vi "EV3_Python.vi"() -> ()   [LabVIEW 2018]
panel:
  in  "Tab Control":enum32{"Connect", "Python"}(tab)
  in  "EV3 IP Address":string="169.254.90.224"
  in  "Ping":bool
  out "Success?":bool
  in  "SSH":bool
  out "SSH Success?":bool
  in  "Script":string="from pybricks import ev3brick as brick\nfrom pybricks.ev3devices import Motor, TouchSensor, ColorSensor,InfraredSensor, UltrasonicSensor, GyroSensor\n\nfrom pybricks.parameters import Port, Stop, Direction, Button, Color, Align\n\nfrom pybricks.tools import wait, StopWatch\n\nexample_motor = Motor (Port.A)"
  out "Console":string
  in  "Help Button":bool
  in  "Run DIrect":bool
  in  "Ctrl C":bool
  in  "Done":bool
  # "Steps:\nGet EV3Dev running\n0. go to https://education.lego.com/en-us/support/mindstorms-ev3/python-for-ev3\n1. burn an SDCard\n2. turn on EV3 with card in\n3. connect to PC\n4. go to Wireless and Networks\n       to All Network Cinnections\n5. select Wired\n6. copy IP address (upper left) \n\nGet Labview running\n7. pip install paramiko  (SSH)\n8. Run this program\n9. hit ping to make sure it is there\n10. hit SSH In\n11. start python"
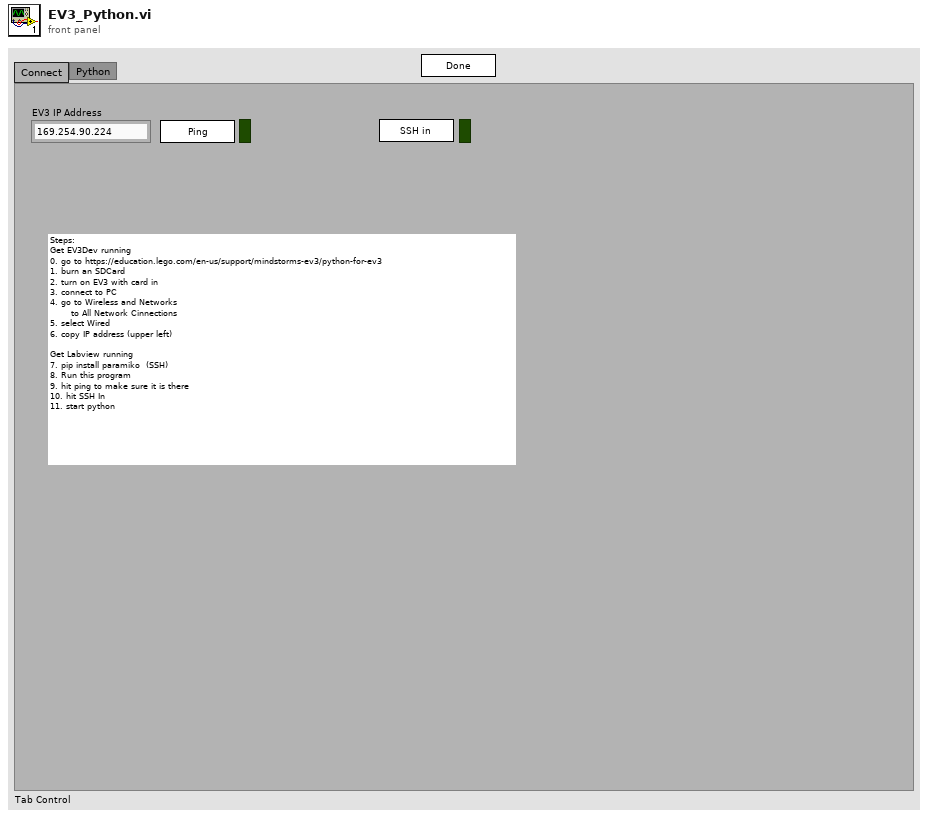
[diagram p1: front panel]
types:
  T1 = typedef "eventvkey.ctl" = enum16{"ASCII", "Enter", "Return", "Shift", "Ctrl", "Alt", "Cmd", "Opt", "Caps", "NumLock", "Clear", "Break", "Up", "Down", "Left", "Right", "Insert", "Delete", "Home", "End", "PageUp", "PageDown", "Escape", "Help", "Pause", "ScrollLock", "F1", "F2", "F3", "F4", "F5", "F6", "F7", "F8", "F9", "F10", "F11", "F12", "F13", "F14", "F15", "F16", "F17", "F18", "F19", "F20", "F21", "F22", "F23", "F24", "Play", "VolumeUp", "VolumeDown", "Mute", "Two Byte Char"}
  T2 = cluster{"Shift":bool, "Ctrl":bool, "Alt":bool, "Cmd":bool, "Opt":bool}
  T3 = cluster{"Char":i16, "VKey":T1, "ScanCode":i16, "Mods":cluster{"Num Pad":bool, "Menu Key":bool}, "PlatMods":cluster{"Shift":bool, "Ctrl":bool, "Alt":bool, "Cmd":bool, "Opt":bool}, "FocusObj":refnum<vi>}
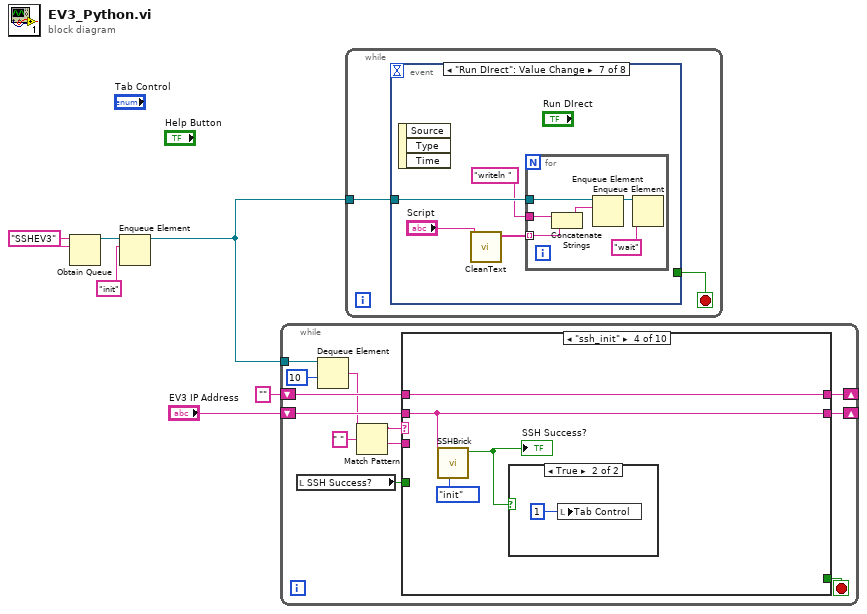
[diagram p0: block diagram]
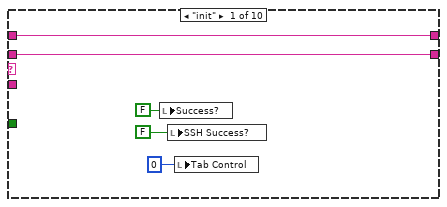
[diagram p2: hidden frame]
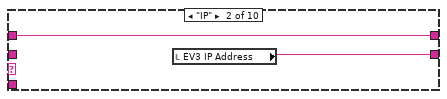
[diagram p3: hidden frame]
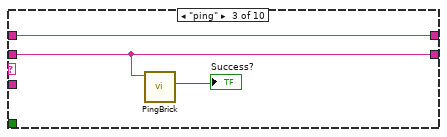
[diagram p4: hidden frame]
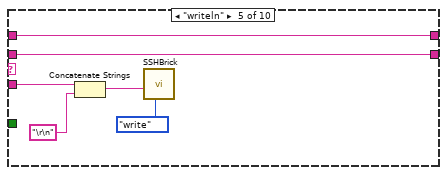
[diagram p6: hidden frame]
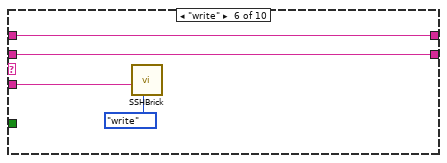
[diagram p7: hidden frame]
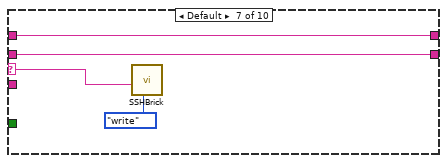
[diagram p8: hidden frame]
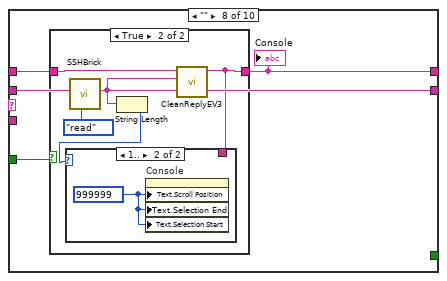
[diagram p9: hidden frame]
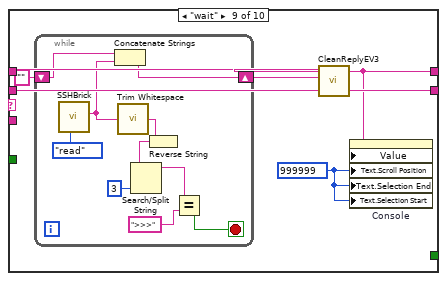
[diagram p12: hidden frame]
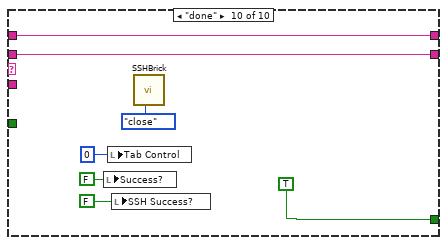
[diagram p13: hidden frame]
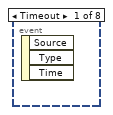
[diagram p14: hidden frame]
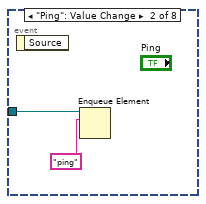
[diagram p15: hidden frame]
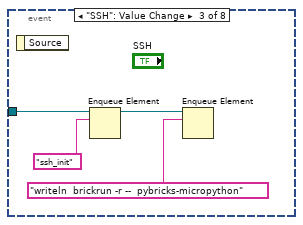
[diagram p16: hidden frame]
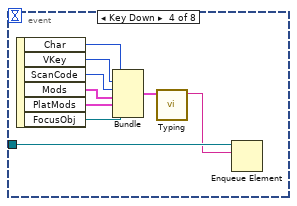
[diagram p17: hidden frame]
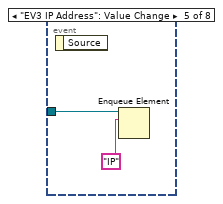
[diagram p18: hidden frame]
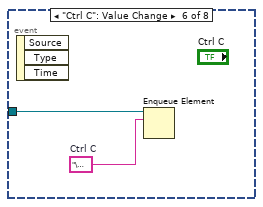
[diagram p19: hidden frame]
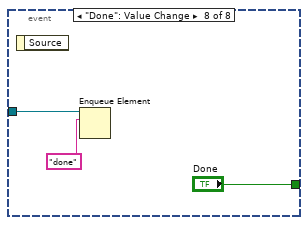
[diagram p20: hidden frame]
diagram:
  w4 = "SSHEV3" ("name (unnamed)")
  n1 = Obtain Queue(name (unnamed)=w4, element data type=w4) -> (queue out=w6:refnum<queue>)  [unwired: 3 in, 2 out]
  n2 = Enqueue Element(queue=w6, element="init") -> (queue out=w3:refnum<queue>)  [unwired: 2 in, 2 out]
  n3 = while {
    tunnel: w3 -> [w18]
    shift-right: [w15] -> _
    shift-left: "EV3 IP Address" -> [w16]
    shift-right: [w13] -> _
    shift-left: "" -> [w14]
    stop <- w17 stop-if-true
    n4 = local read "SSH Success?"() -> (w7:bool)
    n5 = Dequeue Element(queue=w18, timeout in ms (-1)=10) -> (element=w10:string)  [unwired: 1 in, 3 out]
    n6 = Match Pattern(string=w10, regular expression=" ") -> (before substring=w9:string, after substring=w8:string)  [unwired: 1 in, 2 out]
    n7 = case shown="\"ssh_init\"" w9 {
      selector: w9 -> [_ _ _ _ _ _ w44 _ _ _]
      tunnel: [_ _ _ _ _ _ _ _ _ TRUE] -> w17
      tunnel: w16 -> [w23 _ w27 w30 w38 w42 w46 w51 w64 w80]
      tunnel: [w23 w25 w27 w30 w38 w42 w46 w51 w64 w80] -> w15
      tunnel: w14 -> [w22 w24 w26 w32 w39 w43 w47 w50 w59 w79]
      tunnel: [w22 w24 w26 w32 w39 w43 w47 w49 w60 w79] -> w13
      tunnel: w8 -> [_ _ _ _ w34 w40 _ _ _ _]
      tunnel: w7 -> [_ _ _ _ _ _ _ w48 _ _]
      frame "init" {
        n8 = local write "Success?"(FALSE ("Success?")) -> ()
        n9 = local write "SSH Success?"(FALSE ("Success?")) -> ()
        n10 = local write "Tab Control"(0 ("timeout in ms (-1)")) -> ()
      }
      frame "IP" {
        n11 = local read "EV3 IP Address"() -> (w25:string)
      }
      frame "ping" {
        n12 = call "PingBrick.vi"("EV3 IP Address"=w27) -> ("success"=→"Success?":bool)  [unwired: 9 in, 1 out]
      }
      frame "ssh_init" {
        n13 = call "SSHBrick.vi"("Task"=enum16{"init", "read", "write", "close"}."init", "EV3 IP Address"=w30) -> ("Connected?"=w29:bool)  [unwired: 8 in, 1 out]
        "SSH Success?" <- w29
        n14 = case shown="True" w29 {
          frame False {
          }
          frame True {
            n15 = local write "Tab Control"(1 ("timeout in ms (-1)")) -> ()
          }
        }
      }
      frame "writeln" {
        n16 = Concatenate Strings(w34, "\r\n" ("regular expression")) -> (w35:string)
        n17 = call "SSHBrick.vi"("Task"=enum16{"init", "read", "write", "close"}."write", "Text to write"=w35) -> ()  [unwired: 8 in, 2 out]
      }
      frame "write" {
        n18 = call "SSHBrick.vi"("Task"=enum16{"init", "read", "write", "close"}."write", "Text to write"=w40) -> ()  [unwired: 8 in, 2 out]
      }
      frame Default {
        n19 = call "SSHBrick.vi"("Task"=enum16{"init", "read", "write", "close"}."write", "Text to write"=w44) -> ()  [unwired: 8 in, 2 out]
      }
      frame "" {
        n20 = case shown="True" w48 {
          tunnel: w50 -> [w52 w57]
          tunnel: [w52 w53] -> w49
          frame False {
          }
          frame True {
            n21 = call "SSHBrick.vi"("Task"=enum16{"init", "read", "write", "close"}."read") -> ("text read"=w55:string)  [unwired: 9 in, 1 out]
            n22 = String Length(string=w55) -> (length=w54:i32)
            n23 = call "CleanReplyEV3.vi"("text read"=w55, "Console in"=w57) -> ("String out"=w53:string)  [unwired: 9 in]
            n24 = case shown="1.." w54 {
              tunnel: w53 -> [_ _]
              frame 0, Default {
              }
              frame 1.. {
                w58 = u32 999999 ("Text.Scroll Position")
                n25 = property on="Console" class="Str"("Text.Scroll Position"=w58, "Text.Selection End"=w58, "Text.Selection Start"=w58) -> ()  [unwired: 2 in, 2 out]
              }
            }
          }
        }
        "Console" <- w49
      }
      frame "wait" {
        w61 = u32 999999 ("Text.Scroll Position")
        n26 = while {
          shift-right: [w72] -> w63
          shift-left: "" -> [w73]
          stop <- w65 stop-if-true
          n27 = call "SSHBrick.vi"("Task"=enum16{"init", "read", "write", "close"}."read") -> ("text read"=w66:string)  [unwired: 9 in, 1 out]
          n28 = Concatenate Strings(w73, w66) -> (w72:string)
          n29 = call <vilib>:"Trim Whitespace.vi"("string"=w66) -> ("trimmed string"=w71:string)  [unwired: 1 in]
          n30 = Reverse String(1:w71) -> (0:w70:string)
          n31 = Search/Split String(string=w70, offset (0)=3) -> (substring before match=w67:string)  [unwired: 1 in, 2 out]
          n32 = Equal?(x=w67, y=">>>") -> (x = y?=w65:bool)
        }
        n33 = call "CleanReplyEV3.vi"("text read"=w63, "Console in"=w59) -> ("String out"=w60:string)  [unwired: 9 in]
        n34 = property on="Console" class="Str"("Value"=w60, "Text.Scroll Position"=w61, "Text.Selection End"=w61, "Text.Selection Start"=w61) -> ()  [unwired: 2 in, 2 out]
      }
      frame "done" {
        n35 = local write "Success?"(FALSE ("Success?")) -> ()
        n36 = local write "Tab Control"(0 ("timeout in ms (-1)")) -> ()
        n37 = local write "SSH Success?"(FALSE ("Success?")) -> ()
        n38 = call "SSHBrick.vi"("Task"=enum16{"init", "read", "write", "close"}."close") -> ()  [unwired: 9 in, 2 out]
      }
    }
  }
  n39 = while {
    tunnel: w3 -> [w83]
    stop <- w82 stop-if-true
    n40 = event shown="[6] \"Run DIrect\": Value Change" {
      selector: _ -> [_ _ _ _ _ _ _ _]
      dyn-events: _ -> [_ _ _ _ _ _ _ _]
      timeout: _ -> [_ _ _ _ _ _ _ _]
      tunnel: w83 -> [_ w84 w88 w98 w99 w101 w106 w114]
      tunnel: [_ _ _ _ _ _ _ "Done"] -> w82
      event Timeout {
        n41 = event-data() -> ()  [unwired: 1 in, 3 out]
      }
      event "Ping": Value Change {
        n42 = event-data() -> ()  [unwired: 1 in, 1 out]
        n43 = Enqueue Element(queue=w84, element="ping") -> ()  [unwired: 2 in, 3 out]
      }
      event "SSH": Value Change {
        n44 = event-data() -> ()  [unwired: 1 in, 1 out]
        n45 = Enqueue Element(queue=w88, element="ssh_init") -> (queue out=w87:refnum<queue>)  [unwired: 2 in, 2 out]
        n46 = Enqueue Element(queue=w87, element="writeln  brickrun -r --  pybricks-micropython") -> ()  [unwired: 2 in, 3 out]
      }
      event Key Down {
        n47 = event-data() -> ("Char"=w97:i16, "VKey"=w96:T1, "ScanCode"=w95:i16, "Mods"=w94:cluster{"Num Pad":bool, "Menu Key":bool}, "PlatMods"=w93:T2, "FocusObj"=w92:refnum<vi>)  [unwired: 1 in]
        n48 = Bundle("Char"=w97, "VKey"=w96, "ScanCode"=w95, "Mods"=w94, "PlatMods"=w93, "FocusObj"=w92) -> (w91:T3)  [unwired: 1 in]
        n49 = call "Typing.vi"("Cluster"=w91) -> ("string"=w90:string)  [unwired: 8 in, 2 out]
        n50 = Enqueue Element(queue=w98, element=w90) -> ()  [unwired: 2 in, 3 out]
      }
      event "EV3 IP Address": Value Change {
        n51 = event-data() -> ()  [unwired: 1 in, 1 out]
        n52 = Enqueue Element(queue=w99, element="IP") -> ()  [unwired: 2 in, 3 out]
      }
      event "Ctrl C": Value Change {
        w102 = "\u0003"  # Ctrl C
        n53 = event-data() -> ()  [unwired: 1 in, 3 out]
        n54 = Enqueue Element(queue=w101, element=w102) -> ()  [unwired: 2 in, 3 out]
      }
      event "Run DIrect": Value Change {
        n55 = event-data() -> ()  [unwired: 1 in, 3 out]
        n56 = call "CleanText.vi"("Script"="Script") -> ("Array"=w104:string[])  [unwired: 10 in]
        n57 = for {
          tunnel: w106 -> [w112]
          tunnel: w104 -> [w111] mode=indexing
          tunnel: "writeln " ("format string") -> [w110]
          n58 = Concatenate Strings(w110, w111) -> (w109:string)
          n59 = Enqueue Element(queue=w112, element=w109) -> (queue out=w108:refnum<queue>)  [unwired: 2 in, 2 out]
          n60 = Enqueue Element(queue=w108, element="wait" ("format string")) -> ()  [unwired: 2 in, 3 out]
        }
      }
      event "Done": Value Change {
        n61 = event-data() -> ()  [unwired: 1 in, 1 out]
        n62 = Enqueue Element(queue=w114, element="done") -> ()  [unwired: 2 in, 3 out]
      }
    }
  }
